vi "StepperMotorController.vi"() -> ()   [LabVIEW 2013]
doc: "This example shows how to use the Arduino Stepper Motor API. The fritzing diagram shows use with the EasyStepper 4.3 or 4.4 motor controller."
uses:
  <vilib>/LabVIEW Interface for Arduino/Type Defs/Pin Mode.ctl
  <vilib>/LabVIEW Interface for Arduino/LabVIEW Interface for Arduino.lvlib
panel:
  in  "Direction":u8=1 max=1
  in  "Enable":u8=1 max=1
  in  "Stop":bool
  in  "Stepper #":u8=1
  in  "OK Button":bool
  in  "Set Acceleration (0 to disable)":i16
  in  "# of Steps to Move":i16
  in  "Set Speed (Steps per Second)":i16=100 min=0 max=9000 step=1
  out "Steps Remaining?":bool
  in  "Dial":i16(knob) scale=0.0..200.0
  in  "error in":errorcluster
  # "Preset Movement"
  # "Interactive Movement"
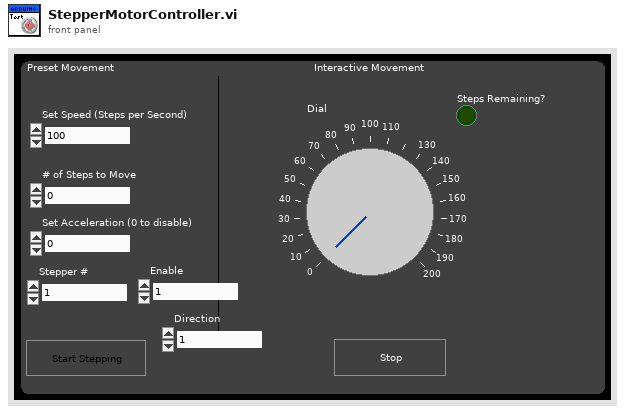
[diagram p1: front panel]
types:
  T1 = typedef "LabVIEW Interface for Arduino.lvlib/Pin Mode.ctl" = enum8{"Input", "Output"}
  T2 = typedef "LabVIEW Interface for Arduino.lvlib/Arduino Resource.ctl" = cluster{"VISA resource":refnum<visa-resource-name>, "Board Type":T3, "Connection Type":enum8{"USB / Serial"}, "Bytes Per Packet (15)":u8}
  T3 = typedef "LabVIEW Interface for Arduino.lvlib/Board Type.ctl" = enum16{"Uno", "Dimuelanove w/Atmega 328", "Mega 2560"}
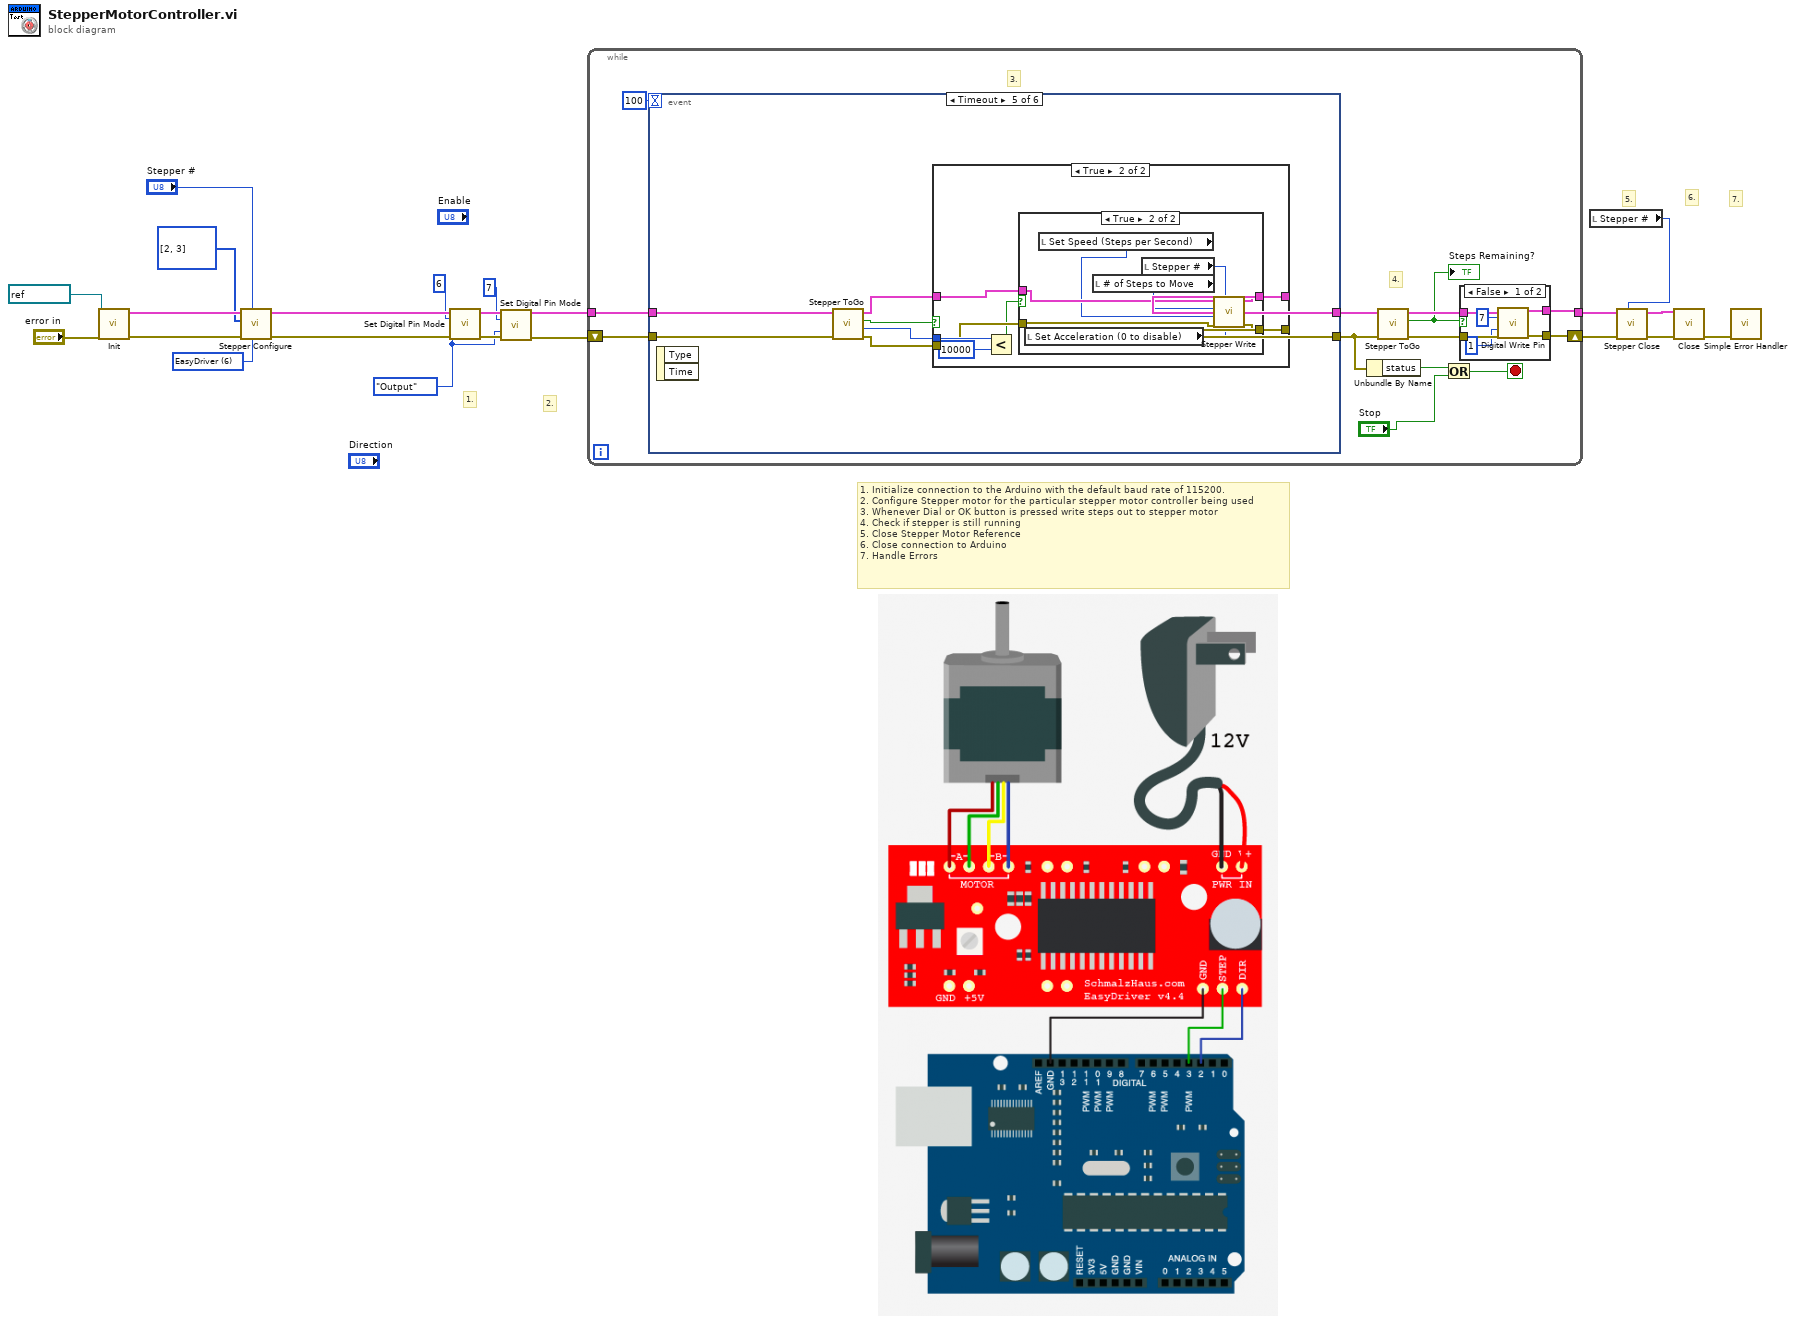
[diagram p0: block diagram]
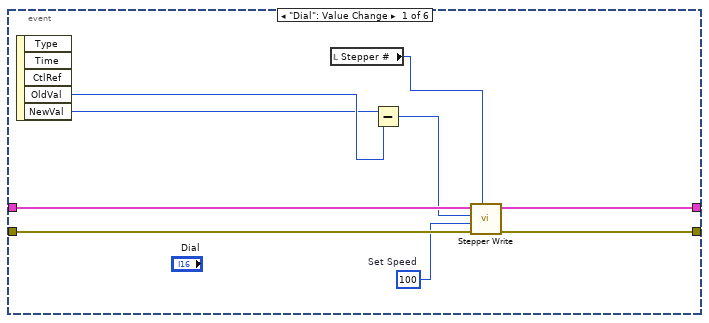
[diagram p3: hidden frame]
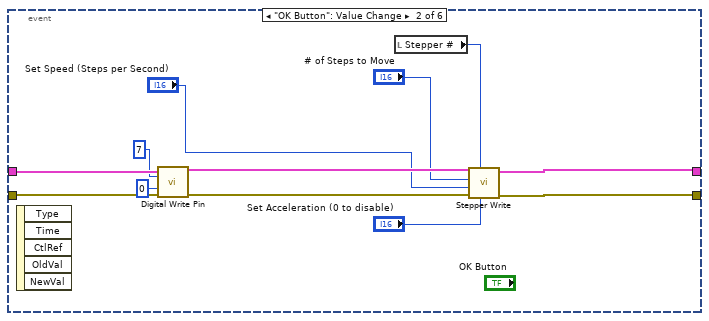
[diagram p4: hidden frame]
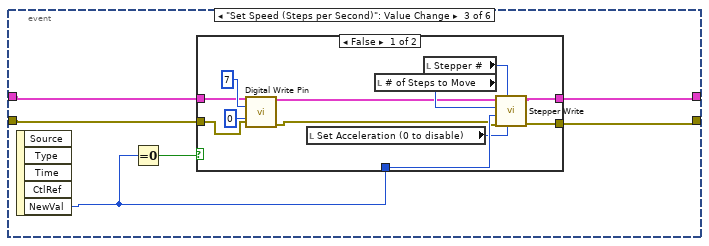
[diagram p5: hidden frame]
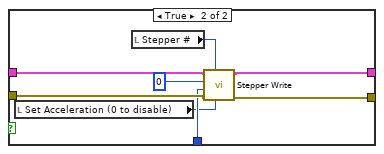
[diagram p6: hidden frame]
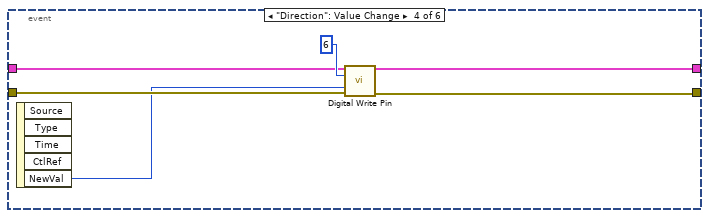
[diagram p7: hidden frame]
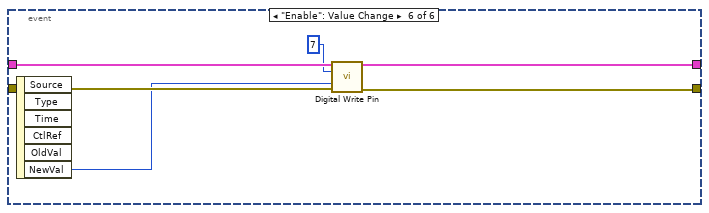
[diagram p10: hidden frame]
diagram:
  w1 = u8 6 items=["2 Wire (Pulse & Direction)"=1, "2 Wire"=2, "4 Wire"=4, "EasyDriver"=6, "AF Motor Shield (Stepper 1 & 2 Only)"=5] ("Control Method")
  w4 = Pin_Mode."Output" ("Pin Mode (Input)")
  # "7."
  # "6."
  # "5."
  # "2."
  # "1."
  # "1. Initialize connection to the Arduino with the default baud rate of 115200.\n2. Configure Stepper motor for the particular stepper motor controller being used\n3. Whenever Dial or OK button is pressed write steps out to stepper motor\n4. Check if stepper is still running\n5. Close Stepper Motor Reference \n6. Close connection to Arduino\n7. Handle Errors"
  n1 = call <vilib>:"Init.vi"("VISA resource"=refnum<visa-resource-name> "COM8", "error in"="error in") -> ("Arduino Resource"=w16:T2, "error out"=w15:errorcluster)  [unwired: 16 in]
  n2 = call <vilib>:"Stepper Configure.vi"("Control Method"=w1, "Stepper #"="Stepper #", "error in"=w15, "Stepper Pins"=u8[] [2, 3], "Arduino Resource"=w16) -> ("error out"=w12:errorcluster, "Arduino Resource Out"=w11:T2)  [unwired: 5 in]
  n3 = call <vilib>:"Set Digital Pin Mode.vi"("Arduino Resource"=w11, "Digital I/O Pin"=u8 6, "Pin Mode (Input)"=w4, "error in"=w12) -> ("Arduino Resource"=w6:T2, "error out"=w9:errorcluster)  [unwired: 10 in]
  n4 = call <vilib>:"Set Digital Pin Mode.vi"("Arduino Resource"=w6, "Digital I/O Pin"=u8 7, "Pin Mode (Input)"=w4, "error in"=w9) -> ("Arduino Resource"=w7:T2, "error out"=w8:errorcluster)  [unwired: 10 in]
  n5 = while {
    tunnel: w7 -> [w34]
    tunnel: [w26] -> w21
    shift-right: [w24] -> w20
    shift-left: w8 -> [w35]
    stop <- w32 stop-if-true
    # "4."
    # "3."
    n6 = event shown="[4] Timeout" {
      selector: _ -> [_ _ _ _ _ _]
      dyn-events: _ -> [_ _ _ _ _ _]
      timeout: 100 -> [_ _ _ _ _ _]
      tunnel: w35 -> [w52 w62 w69 w94 w103 w128]
      tunnel: w34 -> [w51 w64 w70 w95 w104 w129]
      tunnel: [w50 w58 w67 w93 w98 w127] -> w30
      tunnel: [w49 w57 w68 w92 w97 w126] -> w29
      event "Dial": Value Change {
        w46 = i16 100  # Set Speed
        n7 = event-data() -> ("OldVal"=w48:i16, "NewVal"=w47:i16)  [unwired: 1 in, 3 out]
        n8 = local read "Stepper #"() -> (w44:u8)
        n9 = Subtract(x=w47, y=w48) -> (x-y=w45:i16)
        n10 = call <vilib>:"Stepper Write.vi"("Stepper #"=w44, "error in"=w52, "Set Speed (Steps per Second)"=w46, "# of Steps to Move"=w45, "Arduino Resource"=w51) -> ("error out"=w49:errorcluster, "Arduino Resource Out"=w50:T2)  [unwired: 5 in]
      }
      event "OK Button": Value Change {
        n11 = event-data() -> ()  [unwired: 1 in, 5 out]
        n12 = call <vilib>:"Digital Write Pin.vi"("Arduino Resource"=w64, "Digital I/O Pin (0)"=u8 7, "Value (0)"=u8 0, "error in"=w62) -> ("Arduino Resource"=w63:T2, "error out"=w61:errorcluster)  [unwired: 10 in]
        n13 = local read "Stepper #"() -> (w54:u8)
        n14 = call <vilib>:"Stepper Write.vi"("Set Acceleration (0 to disable)"="Set Acceleration (0 to disable)", "Stepper #"=w54, "error in"=w61, "Set Speed (Steps per Second)"="Set Speed (Steps per Second)", "# of Steps to Move"="# of Steps to Move", "Arduino Resource"=w63) -> ("error out"=w57:errorcluster, "Arduino Resource Out"=w58:T2)  [unwired: 4 in]
      }
      event "Set Speed (Steps per Second)": Value Change {
        n15 = event-data() -> ("NewVal"=w66:i16)  [unwired: 1 in, 4 out]
        n16 = Equal To 0?(x=w66) -> (x = 0?=w65:bool)
        n17 = case shown="False" w65 {
          tunnel: w70 -> [w74 w89]
          tunnel: w69 -> [w73 w88]
          tunnel: [w81 w87] -> w68
          tunnel: [w80 w86] -> w67
          tunnel: w66 -> [w79 w85]
          frame False {
            n18 = call <vilib>:"Digital Write Pin.vi"("Arduino Resource"=w74, "Digital I/O Pin (0)"=u8 7, "Value (0)"=u8 0, "error in"=w73) -> ("Arduino Resource"=w71:T2, "error out"=w72:errorcluster)  [unwired: 10 in]
            n19 = local read "Set Acceleration (0 to disable)"() -> (w78:i16)
            n20 = local read "# of Steps to Move"() -> (w77:i16)
            n21 = local read "Stepper #"() -> (w82:u8)
            n22 = call <vilib>:"Stepper Write.vi"("Set Acceleration (0 to disable)"=w78, "Stepper #"=w82, "error in"=w72, "Set Speed (Steps per Second)"=w79, "# of Steps to Move"=w77, "Arduino Resource"=w71) -> ("error out"=w81:errorcluster, "Arduino Resource Out"=w80:T2)  [unwired: 4 in]
          }
          frame True {
            n23 = local read "Set Acceleration (0 to disable)"() -> (w84:i16)
            n24 = local read "Stepper #"() -> (w90:u8)
            n25 = call <vilib>:"Stepper Write.vi"("Set Acceleration (0 to disable)"=w84, "Stepper #"=w90, "error in"=w88, "Set Speed (Steps per Second)"=w85, "# of Steps to Move"=i16 0, "Arduino Resource"=w89) -> ("error out"=w87:errorcluster, "Arduino Resource Out"=w86:T2)  [unwired: 4 in]
          }
        }
      }
      event "Direction": Value Change {
        n26 = event-data() -> ("NewVal"=w91:u8)  [unwired: 1 in, 4 out]
        n27 = call <vilib>:"Digital Write Pin.vi"("Arduino Resource"=w95, "Digital I/O Pin (0)"=u8 6, "Value (0)"=w91, "error in"=w94) -> ("Arduino Resource"=w93:T2, "error out"=w92:errorcluster)  [unwired: 10 in]
      }
      event Timeout {
        n28 = event-data() -> ()  [unwired: 1 in, 2 out]
        n29 = call <vilib>:"Stepper ToGo.vi"("error in"=w103, "Arduino Resource"=w104) -> ("error out"=w99:errorcluster, "Steps remaining"=w101:u16, "Steps Remaining?"=w102:bool, "Arduino Resource Out"=w100:T2)  [unwired: 6 in]
        n30 = case shown="True" w102 {
          tunnel: w101 -> [_ w113]
          tunnel: w100 -> [w106 w110]
          tunnel: w99 -> [w105 w111]
          tunnel: [w106 w109] -> w98
          tunnel: [w105 w108] -> w97
          frame False {
          }
          frame True {
            n31 = Less?(x=w113, y=u16 10000) -> (x < y?=w107:bool)
            n32 = case shown="True" w107 {
              tunnel: w111 -> [w114 w120]
              tunnel: w110 -> [w115 w119]
              tunnel: [w115 w118] -> w109
              tunnel: [w114 w117] -> w108
              frame False {
              }
              frame True {
                n33 = local read "Set Acceleration (0 to disable)"() -> (w122:i16)
                n34 = local read "Set Speed (Steps per Second)"() -> (w116:i16)
                n35 = local read "# of Steps to Move"() -> (w121:i16)
                n36 = local read "Stepper #"() -> (w123:u8)
                n37 = call <vilib>:"Stepper Write.vi"("Set Acceleration (0 to disable)"=w122, "Stepper #"=w123, "error in"=w120, "Set Speed (Steps per Second)"=w116, "# of Steps to Move"=w121, "Arduino Resource"=w119) -> ("error out"=w117:errorcluster, "Arduino Resource Out"=w118:T2)  [unwired: 4 in]
              }
            }
          }
        }
      }
      event "Enable": Value Change {
        n38 = event-data() -> ("NewVal"=w125:u8)  [unwired: 1 in, 5 out]
        n39 = call <vilib>:"Digital Write Pin.vi"("Arduino Resource"=w129, "Digital I/O Pin (0)"=u8 7, "Value (0)"=w125, "error in"=w128) -> ("Arduino Resource"=w127:T2, "error out"=w126:errorcluster)  [unwired: 10 in]
      }
    }
    n40 = Unbundle By Name(w29) -> ("status"=w31:bool)
    n41 = call <vilib>:"Stepper ToGo.vi"("error in"=w29, "Arduino Resource"=w30) -> ("error out"=w25:errorcluster, "Steps Remaining?"=w23:bool, "Arduino Resource Out"=w27:T2)  [unwired: 6 in, 1 out]
    "Steps Remaining?" <- w23
    n42 = Or(x=w31, y="Stop") -> (x .or. y?=w32:bool)
    n43 = case shown="False" w23 {
      tunnel: w27 -> [w41 w43]
      tunnel: [w40 w43] -> w26
      tunnel: w25 -> [w39 w42]
      tunnel: [w38 w42] -> w24
      frame False {
        n44 = call <vilib>:"Digital Write Pin.vi"("Arduino Resource"=w41, "Digital I/O Pin (0)"=u8 7, "Value (0)"=u8 1, "error in"=w39) -> ("Arduino Resource"=w40:T2, "error out"=w38:errorcluster)  [unwired: 10 in]
      }
      frame True {
      }
    }
  }
  n45 = local read "Stepper #"() -> (w14:u8)
  n46 = call <vilib>:"Stepper Close.vi"("Stepper #"=w14, "error in"=w20, "Arduino Resource"=w21) -> ("error out"=w19:errorcluster, "Arduino Resource Out"=w18:T2)  [unwired: 7 in]
  n47 = call <vilib>:"Close.vi"("Arduino Resource"=w18, "error in"=w19) -> ("error out"=w22:errorcluster)  [unwired: 13 in]
  n48 = call <vilib>:"Simple Error Handler.vi"("error in (no error)"=w22) -> ()  [unwired: 4 in, 5 out]
